vi "Four 16-bit Ports Digital Output.vi"(2 "Packet":u64, 4 "Four 16-bit DO Ports":T1={"16-Bit DO Port0"="Chassis2/Mod2/DO15:0", "16-Bit DO Port1"="Chassis2/Mod2/DO15:0", "16-Bit DO Port3"="Chassis2/Mod2/DO15:0", "16-Bit DO Port4"="Chassis2/Mod2/DO15:0"}) -> ()   [LabVIEW 2009]
uses:
  <vilib>/eio/EIONode/EIONode.xnode
  <vilib>/rvi/eio/nirviEIOImplementation/nirviEIOImplementation.xnode
  <vilib>/rvi/eio/common/nirviEmuTemplateMethod_noerrors.vi
  <vilib>/rvi/eio/common/nirviEmuClasses.ctl
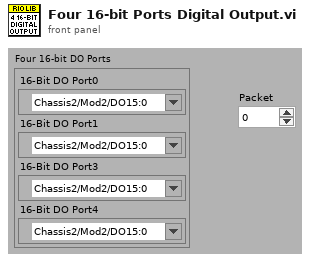
[diagram p1: front panel]
types:
  T1 = cluster{"16-Bit DO Port0":refnum<k21>, "16-Bit DO Port1":refnum<k21>, "16-Bit DO Port3":refnum<k21>, "16-Bit DO Port4":refnum<k21>}
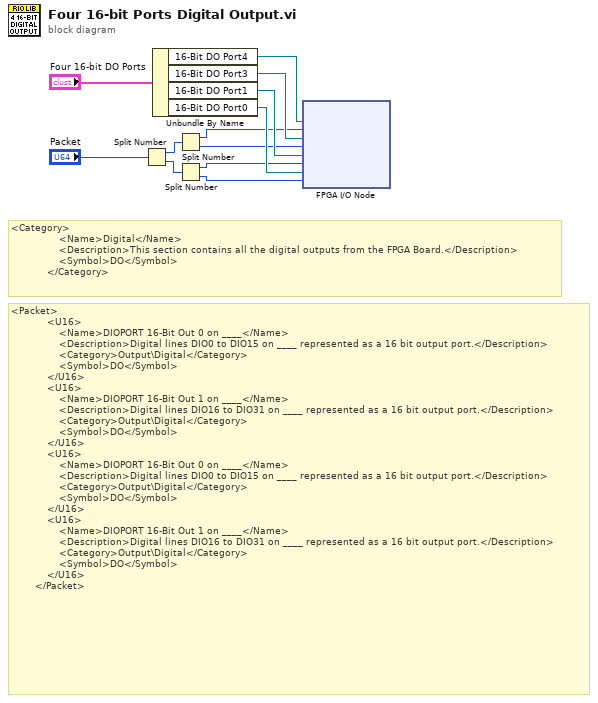
[diagram p0: block diagram]
diagram:
  # "<Packet>\n            <U16>\n                <Name>DIOPORT 16-Bit Out 0 on ____</Name>\n                <Description>Digital lines DIO0 to DIO15 on ____ represented as a 16 bit output port.</Description>\n                <Category>Output\\Digital</Category>\n                <Symbol>DO</Symbol>\n            </U16>\n            <U16>\n                <Name>DIOPORT 16-Bit Out 1 on ____</Name>\n                <Description>Digital lines DIO16 to DIO31 on ____ represented as a 16 bit output port.</Description>\n                <Category>Output\\Digital</Category>\n                <Symbol>DO</Symbol>\n            </U16>\n            <U16>\n                <Name>DIOPORT 16-Bit Out 0 on ____</Name>\n                <Description>Digital lines DIO0 to DIO15 on ____ represented as a 16 bit output port.</Description>\n                <Category>Output\\Digital</Category>\n                <Symbol>DO</Symbol>\n            </U16>\n            <U16>\n                <Name>DIOPORT 16-Bit Out 1 on ____</Name>\n                <Description>Digital lines DIO16 to DIO31 on ____ represented as a 16 bit output port.</Description>\n                <Category>Output\\Digital</Category>\n                <Symbol>DO</Symbol>\n            </U16>\n        </Packet>"
  # "<Category>\n                <Name>Digital</Name>\n                <Description>This section contains all the digital outputs from the FPGA Board.</Description>\n                <Symbol>DO</Symbol>\n            </Category>"
  n1 = Split Number(x="Packet") -> (hi(x)=w4:u32, lo(x)=w12:u32)
  n2 = Unbundle By Name("Four 16-bit DO Ports") -> ("16-Bit DO Port4"=w2:refnum<k21>, "16-Bit DO Port3"=w5:refnum<k21>, "16-Bit DO Port1"=w9:refnum<k21>, "16-Bit DO Port0"=w8:refnum<k21>)
  n3 = Split Number(x=w4) -> (hi(x)=w1:u16, lo(x)=w3:u16)
  n4 = Split Number(x=w12) -> (hi(x)=w7:u16, lo(x)=w6:u16)
  n5 = xnode "FPGA I/O Node"("I/O Item"=w1, "I/O Item"=w3, "I/O Item"=w7, "I/O Item"=w6, "FPGA I/O In"=w2, "FPGA I/O In"=w5, "FPGA I/O In"=w9, "FPGA I/O In"=w8) -> ()  [unwired: 4 out]
